vi "Script Error VI Template with custom data.vi"(4 "Error Code":i32, 5 "Selection Type":T1, 6 "Error Name":string, 7 "Error Arguments Window Ref":refnum<vi>, 8 "error in":errorcluster, 9 "Error Description":string, 10 "Library Path":path, 11 "VI Ref Error in":refnum<vi>) -> (0 "error out":errorcluster, 3 "Custom Error VI Ref":refnum<vi>)   [LabVIEW 2020, in "ConstantErrorsMaker.lvlib"]
uses:
  ConstantErrorsMaker.lvlib
  Selection Type--enum.ctl
  <vilib>/Utility/traverseref.llb/TRef TravTarget.ctl
  <vilib>/Utility/miscctls.llb/LVPositionTypeDef.ctl
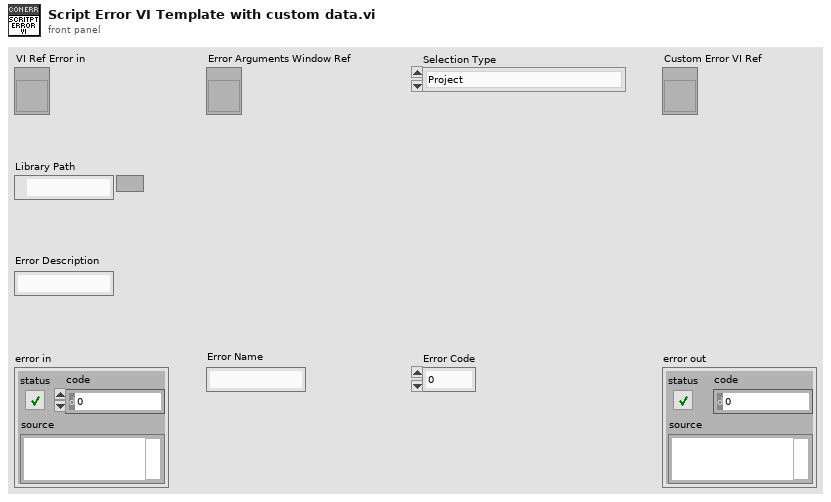
[diagram p1: front panel]
types:
  T1 = typedef "ConstantErrorsMaker.lvlib/Selection Type--enum.ctl" = enum16{"Project", "Library", "Class", "DQMH Singleton", "DQMH Cloneable"}
  T2 = typedef "TRef TravTarget.ctl" = enum16{"FP", "BD", "Other"}
  T3 = typedef "LVPositionTypeDef.ctl" = cluster{"Left":i32, "Top":i32}
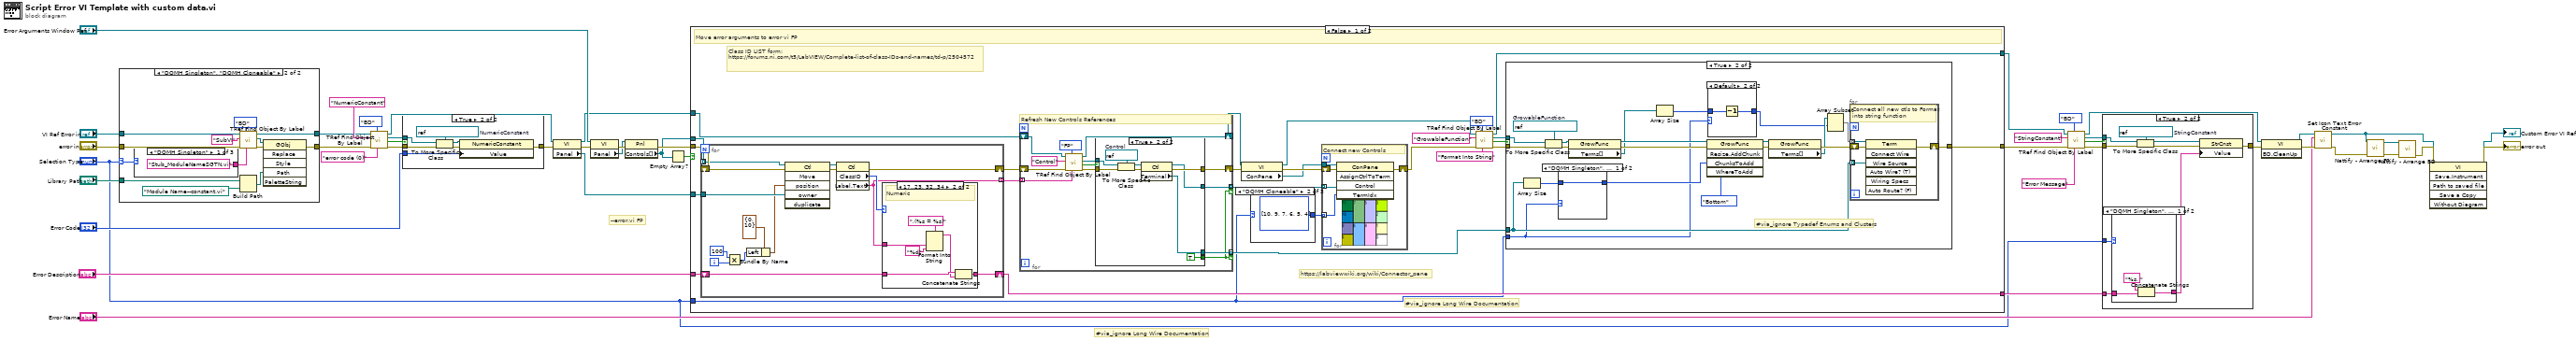
[diagram p0: block diagram]
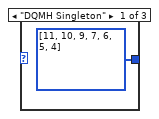
[diagram p2: hidden frame]
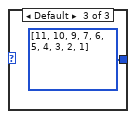
[diagram p3: hidden frame]
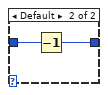
[diagram p6: hidden frame]
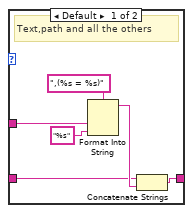
[diagram p8: hidden frame]
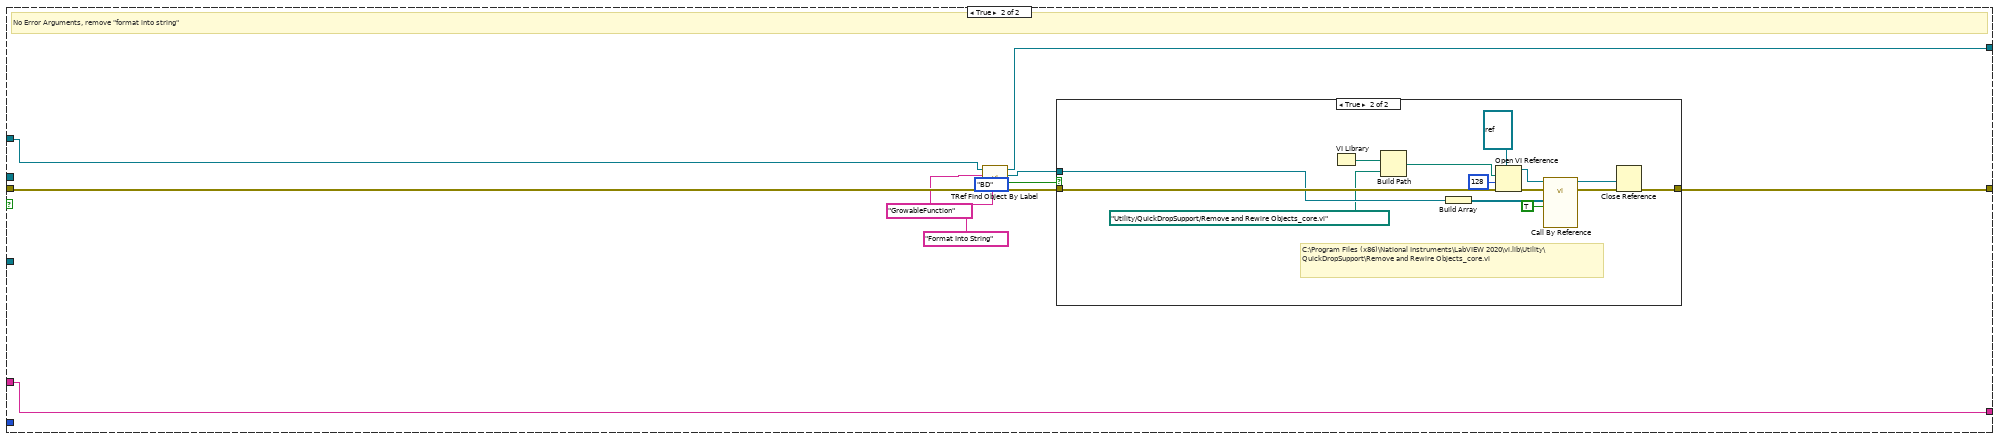
[diagram p9: hidden frame]
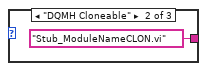
[diagram p15: hidden frame]
diagram:
  # "#via_ignore Long Wire Documentation"
  # "--error.vi FP"
  n1 = case shown="\"DQMH Singleton\", \"DQMH Cloneable\"" "Selection Type" {
    selector: "Selection Type" -> [_ w49]
    tunnel: [w48 w60] -> w33
    tunnel: "error in" -> [w48 w59]
    tunnel: "VI Ref Error in" -> [w47 w52]
    tunnel: [w47 w51] -> w3
    tunnel: "Library Path" -> [_ w50]
    frame Default {
    }
    frame "DQMH Singleton", "DQMH Cloneable" {
      n2 = case shown="\"DQMH Singleton\"" w49 {
        tunnel: ["Stub_ModuleNameSGTN.vi" ("Label") "Stub_ModuleNameCLON.vi" ("Label") _] -> w53
        frame "DQMH Singleton" {
        }
        frame "DQMH Cloneable" {
        }
        frame Default {
        }
      }
      n3 = call <vilib>:"TRef Find Object By Label.vi"("Label"=w53, "Traverse Target"=TRef_TravTarget."BD", "error in (no error)"=w59, "Class Name"="SubVI", "VI Ref"=w52) -> ("error out"=w61:errorcluster, "Found Obj Ref"=w54:refnum<vi>, "dup VI Ref"=w51:refnum<vi>)  [unwired: 3 in, 1 out]
      n4 = Build Path(base path=w50, name or relative path=path "Module Name--constant.vi") -> (appended path=w56:path)
      n5 = invoke class="GObj" method="Replace"(reference=w54, error in=w61, "Path"=w56) -> (error out=w60:errorcluster)  [unwired: 3 in, 5 out]
    }
  }
  n6 = call <vilib>:"TRef Find Object By Label.vi"("Label"="error code (0)", "Traverse Target"=TRef_TravTarget."BD", "error in (no error)"=w33, "Class Name"="NumericConstant", "VI Ref"=w3) -> ("error out"=w46:errorcluster, "Found?"=w28:bool, "Found Obj Ref"=w27:refnum<vi>, "dup VI Ref"=w16:refnum<vi>)  [unwired: 3 in]
  n7 = case shown="True" w28 {
    tunnel: w46 -> [w64 w71]
    tunnel: w27 -> [_ w68]
    tunnel: "Error Code" -> [_ w65]
    tunnel: [w64 w69] -> w41
    frame False {
    }
    frame True {
      w67 = refnum<vi> refnum  # NumericConstant
      n8 = To More Specific Class(target class=w67, reference=w68, error in=w71) -> (specific class reference=w66:refnum<vi>, error out=w70:errorcluster)
      n9 = property class="NumericConstant"(reference=w66, error in=w70, "Value"=w65) -> (error out=w69:errorcluster)  [unwired: 1 out]
    }
  }
  n10 = property class="VI"(reference=w16, error in=w41) -> (reference out=w15:refnum<vi>, error out=w42:errorcluster, "Panel"=w17:refnum<vi>)
  n11 = property class="VI"(reference="Error Arguments Window Ref", error in=w42) -> (error out=w44:errorcluster, "Panel"=w20:refnum<vi>)  [unwired: 1 out]
  n12 = property class="Pnl"(reference=w20, error in=w44) -> (error out=w43:errorcluster, "Controls[]"=w18:refnum<vi>[])  [unwired: 1 out]
  n13 = Empty Array?(array=w18) -> (empty?=w19:bool)
  n14 = case shown="False" w19 {
    tunnel: w43 -> [w97 w198]
    tunnel: w18 -> [w81 _]
    tunnel: w17 -> [w90 _]
    tunnel: [w95 w196] -> w40
    tunnel: "Error Description" -> [w89 w195]
    tunnel: [w88 w195] -> w12
    tunnel: w15 -> [w78 w191]
    tunnel: [w87 w189] -> w14
    tunnel: "Selection Type" -> [w72 _]
    frame False {
      # "#via_ignore Long Wire Documentation"
      # "https://labviewwiki.org/wiki/Connector_pane"
      # "Class ID LIST form:\nhttps://forums.ni.com/t5/LabVIEW/Complete-list-of-class-IDs-and-names/td-p/2504572"
      # "Move error arguments to error vi FP"
      n15 = for {
        tunnel: w81 -> [w167] mode=indexing
        tunnel: w90 -> [w166]
        shift-right: [w168] -> w94
        shift-left: w97 -> [w170]
        shift-right: [w161] -> w88
        shift-left: w89 -> [w162]
        tunnel: [w160] -> w80 mode=indexing
        i -> [w158]
        n16 = Multiply(x=100, y=w158) -> (x*y=w157:i32)
        n17 = Bundle By Name(cluster=T3 {"Left"=0, "Top"=10} ("position"), "Left"=w157) -> (w159:T3)
        n18 = invoke class="Ctl" method="Move"(reference=w167, error in=w170, "position"=w159, "owner"=w166) -> (reference out=w164:refnum<vi>, error out=w169:errorcluster)  [unwired: 2 in, 4 out]
        n19 = property class="Ctl"(reference=w164, error in=w169) -> (error out=w168:errorcluster, "ClassID"=w163:u32, "Label.Text"=w160:string)  [unwired: 1 out]
        n20 = case shown="17..23, 32..34" w163 {
          tunnel: w162 -> [w172 w182]
          tunnel: [w173 w181] -> w161
          tunnel: w160 -> [w171 w180]
          frame Default {
            # "Text,path and all the others"
            n21 = Format Into String(format string=",(%s = %s)", w171, "%s" ("string")) -> (resulting string=w174:string)  [unwired: 2 in, 1 out]
            n22 = Concatenate Strings(w172, w174) -> (w173:string)
          }
          frame 17..23, 32..34 {
            # "Numeric"
            n23 = Format Into String(format string=",(%s = %s)", w180, "%d" ("string")) -> (resulting string=w177:string)  [unwired: 2 in, 1 out]
            n24 = Concatenate Strings(w182, w177) -> (w181:string)
          }
        }
      }
      n25 = for {
        tunnel: w80 -> [w142] mode=indexing
        shift-right: [w143] -> w93
        shift-left: w94 -> [w145]
        tunnel: [w138] -> w79 mode=indexing if=w133
        shift-right: [w135] -> w77
        shift-left: w78 -> [w137]
        tunnel: [w134] -> w74 mode=indexing if=w133
        # "Refresh New Controls References"
        n26 = call <vilib>:"TRef Find Object By Label.vi"("Label"=w142, "Traverse Target"=TRef_TravTarget."FP", "error in (no error)"=w145, "Class Name"="Control", "VI Ref"=w137) -> ("error out"=w144:errorcluster, "Found?"=w136:bool, "Found Obj Ref"=w140:refnum<vi>, "dup VI Ref"=w135:refnum<vi>)  [unwired: 3 in]
        n27 = case shown="True" w136 {
          tunnel: w140 -> [_ w152]
          tunnel: [_ w148] -> w138
          tunnel: w144 -> [w146 w155]
          tunnel: [w146 w153] -> w143
          tunnel: [_ TRUE] -> w133
          tunnel: [_ w149] -> w134
          frame False {
          }
          frame True {
            w151 = refnum<vi> refnum  # Control
            n28 = To More Specific Class(target class=w151, reference=w152, error in=w155) -> (specific class reference=w147:refnum<vi>, error out=w154:errorcluster)
            n29 = property class="Ctl"(reference=w147, error in=w154) -> (reference out=w149:refnum<vi>, error out=w153:errorcluster, "Terminal"=w148:refnum<vi>)
          }
        }
      }
      n30 = property class="VI"(reference=w77, error in=w93) -> (reference out=w76:refnum<vi>, error out=w92:errorcluster, "ConPane"=w75:refnum<vi>)
      n31 = case shown="\"DQMH Cloneable\"" w72 {
        tunnel: [i32[] [11, 10, 9, 7, 6, 5, 4] i32[] [10, 9, 7, 6, 5, 4] i32[] [11, 10, 9, 7, 6, 5, 4, 3, 2, 1]] -> w73
        frame "DQMH Singleton" {
        }
        frame "DQMH Cloneable" {
        }
        frame Default {
        }
      }
      n32 = for {
        tunnel: w75 -> [w185]
        shift-right: [w186] -> w91
        shift-left: w92 -> [w187]
        tunnel: w74 -> [w184] mode=indexing
        tunnel: w73 -> [w183] mode=indexing
        # "Connect new Controls"
        n33 = invoke class="ConPane" method="AssignCtrlToTerm"(reference=w185, error in=w187, "Control"=w184, "TermIdx"=w183) -> (error out=w186:errorcluster)  [unwired: 1 in, 4 out]
      }
      n34 = call <vilib>:"TRef Find Object By Label.vi"("Label"="Format Into String", "Traverse Target"=TRef_TravTarget."BD", "error in (no error)"=w91, "Class Name"="GrowableFunction", "VI Ref"=w76) -> ("error out"=w96:errorcluster, "Found?"=w84:bool, "Found Obj Ref"=w83:refnum<vi>, "dup VI Ref"=w87:refnum<vi>)  [unwired: 3 in]
      n35 = case shown="True" w84 {
        tunnel: w96 -> [w101 w122]
        tunnel: w83 -> [_ w116]
        tunnel: [w101 w117] -> w95
        tunnel: w79 -> [_ w106]
        tunnel: w72 -> [_ w102]
        frame False {
        }
        frame True {
          w115 = refnum<vi> refnum  # GrowableFunction
          # "#via_ignore Typedef Enums and Clusters"
          n36 = Array Size(array=w106) -> (size(s)=w113:i32)
          n37 = To More Specific Class(target class=w115, reference=w116, error in=w122) -> (specific class reference=w111:refnum<vi>, error out=w121:errorcluster)
          n38 = case shown="\"DQMH Singleton\", \"DQMH Cloneable\"" w102 {
            tunnel: w113 -> [w126 w128]
            tunnel: [w126 w127] -> w105
            frame "DQMH Singleton", "DQMH Cloneable" {
            }
            frame Default {
              n39 = Decrement(x=w128) -> (x-1=w127:i32)
            }
          }
          n40 = property class="GrowFunc"(reference=w111, error in=w121) -> (reference out=w110:refnum<vi>, error out=w119:errorcluster, "Terms[]"=w109:refnum<vi>[])
          n41 = Array Size(array=w109) -> (size(s)=w104:i32)
          n42 = invoke class="GrowFunc" method="Resize.AddChunk"(reference=w110, error in=w119, "ChunksToAdd"=w105, "WhereToAdd"=enum8{"Bottom", "Top"}."Bottom" ("Where To Add")) -> (reference out=w112:refnum<vi>, error out=w120:errorcluster)  [unwired: 1 in, 3 out]
          n43 = case shown="Default" w102 {
            tunnel: w104 -> [w123 w125]
            tunnel: [w123 w124] -> w103
            frame "DQMH Singleton", "DQMH Cloneable" {
            }
            frame Default {
              n44 = Decrement(x=w125) -> (x-1=w124:i32)
            }
          }
          n45 = property class="GrowFunc"(reference=w112, error in=w120) -> (error out=w118:errorcluster, "Terms[]"=w108:refnum<vi>[])  [unwired: 1 out]
          n46 = Array Subset(array=w108, index=w103) -> (w107:refnum<vi>[])  [unwired: 1 in]
          n47 = for {
            tunnel: w107 -> [w130] mode=indexing
            tunnel: w106 -> [w129] mode=indexing
            shift-right: [w131] -> w117
            shift-left: w118 -> [w132]
            # "Connect all new ctls to Format into string function"
            n48 = invoke class="Term" method="Connect Wire"(reference=w130, error in=w132, "Wire Source"=w129) -> (error out=w131:errorcluster)  [unwired: 4 in, 6 out]
          }
        }
      }
    }
    frame True {
      # "No Error Arguments, remove \"format into string\""
      n49 = call <vilib>:"TRef Find Object By Label.vi"("Label"="Format Into String", "Traverse Target"=TRef_TravTarget."BD", "error in (no error)"=w198, "Class Name"="GrowableFunction", "VI Ref"=w191) -> ("error out"=w197:errorcluster, "Found?"=w190:bool, "Found Obj Ref"=w188:refnum<vi>, "dup VI Ref"=w189:refnum<vi>)  [unwired: 3 in]
      n50 = case shown="True" w190 {
        tunnel: w197 -> [w199 w211]
        tunnel: [w199 w210] -> w196
        tunnel: w188 -> [_ w209]
        frame False {
        }
        frame True {
          # "C:\\Program Files (x86)\\National Instruments\\LabVIEW 2020\\vi.lib\\Utility\\QuickDropSupport\\Remove and Rewire Objects_core.vi"
          n51 = VI Library() -> (path=w203:path)
          n52 = Build Path(base path=w203, name or relative path=path "Utility/QuickDropSupport/Remove and Rewire Objects_core.vi") -> (appended path=w201:path)
          n53 = Build Array(w209) -> (w206:refnum<vi>[])
          n54 = Open VI Reference(type specifier VI Refnum (for type only)=refnum<vi> refnum, vi path=w201, options=128, error in (no error)=w211) -> (vi reference=w207:refnum<vi>, error out=w213:errorcluster)  [unwired: 2 in]
          n55 = call-by-ref "?"(reference=w207, error in=w213, "Clean Wires (T)"=TRUE, "Items to Remove"=w206) -> (reference out=w205:refnum<vi>, error out=w212:errorcluster)  [unwired: 8 in, 2 out]
          n56 = Close Reference(reference=w205, error in (no error)=w212) -> (error out=w210:errorcluster)
        }
      }
    }
  }
  n57 = call <vilib>:"TRef Find Object By Label.vi"("Label"="Error Message", "Traverse Target"=TRef_TravTarget."BD", "error in (no error)"=w40, "Class Name"="StringConstant", "VI Ref"=w14) -> ("error out"=w45:errorcluster, "Found?"=w23:bool, "Found Obj Ref"=w22:refnum<vi>, "dup VI Ref"=w6:refnum<vi>)  [unwired: 3 in]
  n58 = case shown="True" w23 {
    tunnel: w45 -> [w214 w223]
    tunnel: w22 -> [_ w220]
    tunnel: [w214 w221] -> w35
    tunnel: w12 -> [_ w216]
    tunnel: "Selection Type" -> [_ w217]
    frame False {
    }
    frame True {
      w219 = refnum<vi> refnum  # StringConstant
      n59 = case shown="\"DQMH Singleton\", \"DQMH Cloneable\"" w217 {
        tunnel: w216 -> [w225 w227]
        tunnel: [w224 w227] -> w215
        frame "DQMH Singleton", "DQMH Cloneable" {
          n60 = Concatenate Strings("%s, " ("string"), w225) -> (w224:string)
        }
        frame Default {
        }
      }
      n61 = To More Specific Class(target class=w219, reference=w220, error in=w223) -> (specific class reference=w218:refnum<vi>, error out=w222:errorcluster)
      n62 = property class="StrCnst"(reference=w218, error in=w222, "Value"=w215) -> (error out=w221:errorcluster)  [unwired: 1 out]
    }
  }
  n63 = invoke class="VI" method="BD.CleanUp"(reference=w6, error in=w35) -> (reference out=w5:refnum<vi>, error out=w34:errorcluster)  [unwired: 1 in, 1 out]
  n64 = call "Set Icon Text Error Constant.vi"("error in"=w34, "Text"="Error Name", "VI in"=w5) -> ("error out"=w39:errorcluster, "VI out"=w9:refnum<vi>)  [unwired: 7 in]
  n65 = call "Nattify - Arrange FP.vi"("VI in"=w9, "error in"=w39) -> ("VI out"=w10:refnum<vi>, "error out"=w37:errorcluster)  [unwired: 12 in]
  n66 = call "Nattify - Arrange BD.vi"("VI in"=w10, "error in"=w37) -> ("error out"=w36:errorcluster)  [unwired: 13 in]
  n67 = invoke class="VI" method="Save.Instrument"(reference=w9, error in=w36) -> (reference out=→"Custom Error VI Ref":refnum<vi>, error out=→"error out":errorcluster)  [unwired: 4 in, 4 out]
